vi "tsfifo_receive_can_msgs.vi"(7 "error in (no error)":errorcluster caption="错误输入（无错误）", 8 "Read message type":u16(ring) items=["只读取接收报文", "发送报文&接收报文"], 9 "AAPPChannel":u32, 10 "Path":path) -> (0 "error out":errorcluster caption="错误输出", 1 "Return":i32, 2 "ACANMsgBuffer":T1(array[cluster]), 3 "Path output":path)   [LabVIEW 2014]
doc: "Function Introduction :\nReceive FIFO CAN messages\nCall location :\ninput parameter :\nACANBuffers: CAN buffers\nACANBufferSize: can buffer size\nAChn: Channel Index\nARxTx: READ_TX_RX_deF_ARxTx enumeration, if the value is 0, only RX messages are received; if the value is\n1. Receive TX Rx message\nReturn value :\n0: Execution successful\nOther values: Failed"
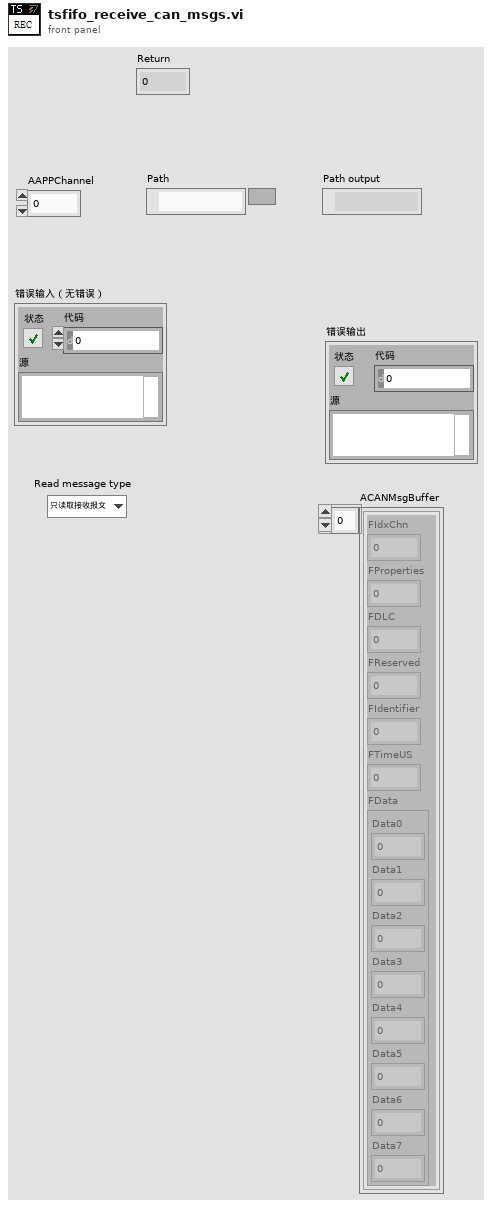
[diagram p1: front panel]
types:
  T1 = cluster{"FIdxChn":u8, "FProperties":u8, "FDLC":u8, "FReserved":u8, "FIdentifier":i32, "FTimeUS":u64, "FData":cluster{"Data0":u8, "Data1":u8, "Data2":u8, "Data3":u8, "Data4":u8, "Data5":u8, "Data6":u8, "Data7":u8}}[]
  T2 = cluster{"FIdxChn":u8, "FProperties":u8, "FDLC":u8, "FReserved":u8, "FIdentifier":i32, "FTimeUS":u64, "FData":cluster{"Data0":u8, "Data1":u8, "Data2":u8, "Data3":u8, "Data4":u8, "Data5":u8, "Data6":u8, "Data7":u8}}
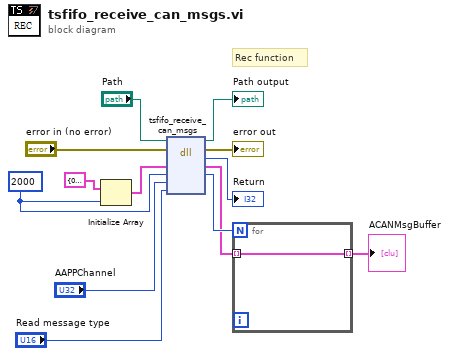
[diagram p0: block diagram]
diagram:
  w1 = 2000 ("维数大小")
  # "Rec function"
  n1 = Initialize Array(T2 {"FIdxChn"=0, "FProperties"=0, "FDLC"=0, "FReserved"=0, "FIdentifier"=0, "FTimeUS"=0, "FData"={"Data0"=0, "Data1"=0, "Data2"=0, "Data3"=0, "Data4"=0, "Data5"=0, "Data6"=0, "Data7"=0}} ("簇"), w1) -> (w13:T1)
  n2 = dll-call lib="PTH2Habs CUsers\nAdministratorDesktopTS_Can通讯PathTSMaster.dll" fn="tsfifo_receive_can_msgs"(path in="Path", error in="error in (no error)", "ACANMsgBuffer"=w13, "ACANMsgBufferSize"=w1, "AChn"="AAPPChannel", "ATxRx"="Read message type") -> (path out=→"Path output":path, error out=→"error out":errorcluster, "tsfifo_receive_can_msgs"=→"Return":i32, "ACANMsgBuffer"=w4:T1, "ACANMsgBufferSize"=w5:i32)  [unwired: 3 in]
  n3 = for {
    N: w5 -> [_]
    tunnel: w4 -> [w14] mode=indexing
    tunnel: [w14] -> w3 mode=indexing
  }
  "ACANMsgBuffer" <- w3
